vi "sort polymorphs.vi"   [LabVIEW 2013]
uses:
  source/tag/count types.vi
  source/tag/index to type.vi
  source/tag/data bus tag description.lvclass
  source/table/data bus values.lvlib
types:
  T1 = typedef "data bus tag description.lvclass/Data Type.ctl" = enum16{"Double", "Single", "I64", "I32", "I16", "I8", "U64", "U32", "U16", "U8", "Boolean", "String", "Array of Double", "Array of Single", "Array of I64", "Array of I32", "Array of I16", "Array of I8", "Array of U64", "Array of U32", "Array of U16", "Array of U8", "Array of Boolean", "Array of String"}
  T2 = cluster{"VIPath":path, "Menu Name":string, "Selector Name":string}[]
  T3 = cluster{"VIPath":path, "Menu Name":string, "Selector Name":string}
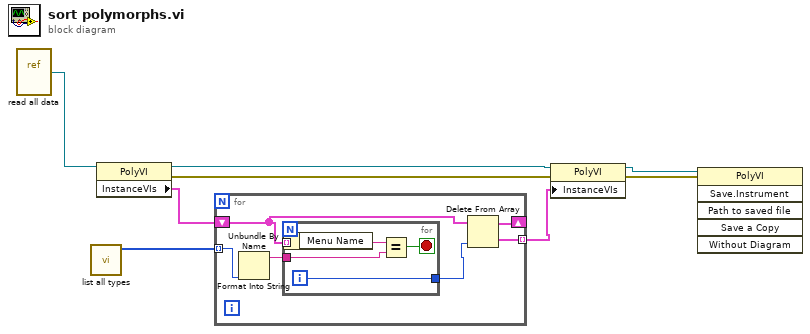
[diagram p0: block diagram]
diagram:
  n1 = vi-ref "read all data.vi"() -> (w1:refnum<vi>)
  n2 = call "list all types.vi"() -> ("all types"=w4:T1[])  [unwired: 11 in]
  n3 = property class="PolyVI"(reference=w1) -> (reference out=w8:refnum<vi>, error out=w5:errorcluster, "InstanceVIs"=w3:T2)  [unwired: 1 in]
  n4 = for {
    tunnel: w4 -> [w14] mode=indexing
    shift-right: [w11] -> _
    shift-left: w3 -> [w12]
    tunnel: [w9] -> w2 mode=indexing
    n5 = Format Into String(w14) -> (resulting string=w13:string)  [unwired: 3 in, 1 out]
    n6 = for {
      tunnel: w12 -> [w19] mode=indexing
      tunnel: w13 -> [w17]
      tunnel: [w15] -> w10
      i -> [w15]
      stop <- w16 stop-if-true
      n7 = Unbundle By Name(w19) -> ("Menu Name"=w18:string)
      n8 = Equal?(x=w18, y=w17) -> (x = y?=w16:bool)
    }
    n9 = Delete From Array(array=w12, index=w10) -> (deleted portion=w9:T3, array with subset deleted=w11:T2)  [unwired: 1 in]
  }
  n10 = property class="PolyVI"(reference=w8, error in=w5, "InstanceVIs"=w2) -> (reference out=w7:refnum<vi>, error out=w6:errorcluster)
  n11 = invoke class="PolyVI" method="Save.Instrument"(reference=w7, error in=w6) -> ()  [unwired: 4 in, 6 out]
